vi "VPD Test Panel.vi"() -> ()   [LabVIEW 2020]
uses:
  Desktop/Vision Point LabVIEW/KYFGLib_lv.lvlib
panel:
  out "Intensity Graph":u16[][](graph)
  out "size(s) 0":i32
  in  "Pixel format":enum16{"Mono8", "Mono10", "Mono12"}(ring)
  in  "Adjust width":bool
  in  "Horizontal Pixel slider":cluster{i64, i64}(slide)={9072, 0} scale=0.0..9072.0
  in  "Height":i64=256
  in  "paramValueName":string
  in  "Boolean":bool=TRUE
  out "paramValue our [Float]":dbl
  out "frame index":i32
  out "buffer size":u64
  out "buffHandle":u32
  in  "Start stream":bool
  in  "Float Value (set)":dbl
  in  "Send command":bool
  in  "Integer Value (set)":i64=1
  out "function return":u32
  out "stringValueOut":string
  out "paramValue out [Int]":i64
  in  "Frame Grabber":bool=TRUE
  in  "Camera":bool
  in  "Set Parameter":string
  in  "Get Parameter":string
  out "Frame Grabber handle":u32=65536 caption="FG handle"
  out "Camera handle":u32
  out "Frame Grabbers":string[](array[string])
  in  "Quit":bool
  out "Last Error":errorcluster
  # "Example Commands:\n\nGet info for device\n0in\n\nGet device status\n0gs\n\nGo to home position (position 0)\n0ho0\n\nGo to position 0\n0ma00000000\n\nGo to position 1\n0ma00000020\n\nGo to position 2\n0ma00000040\n\nGo to position 3\n0ma00000060"
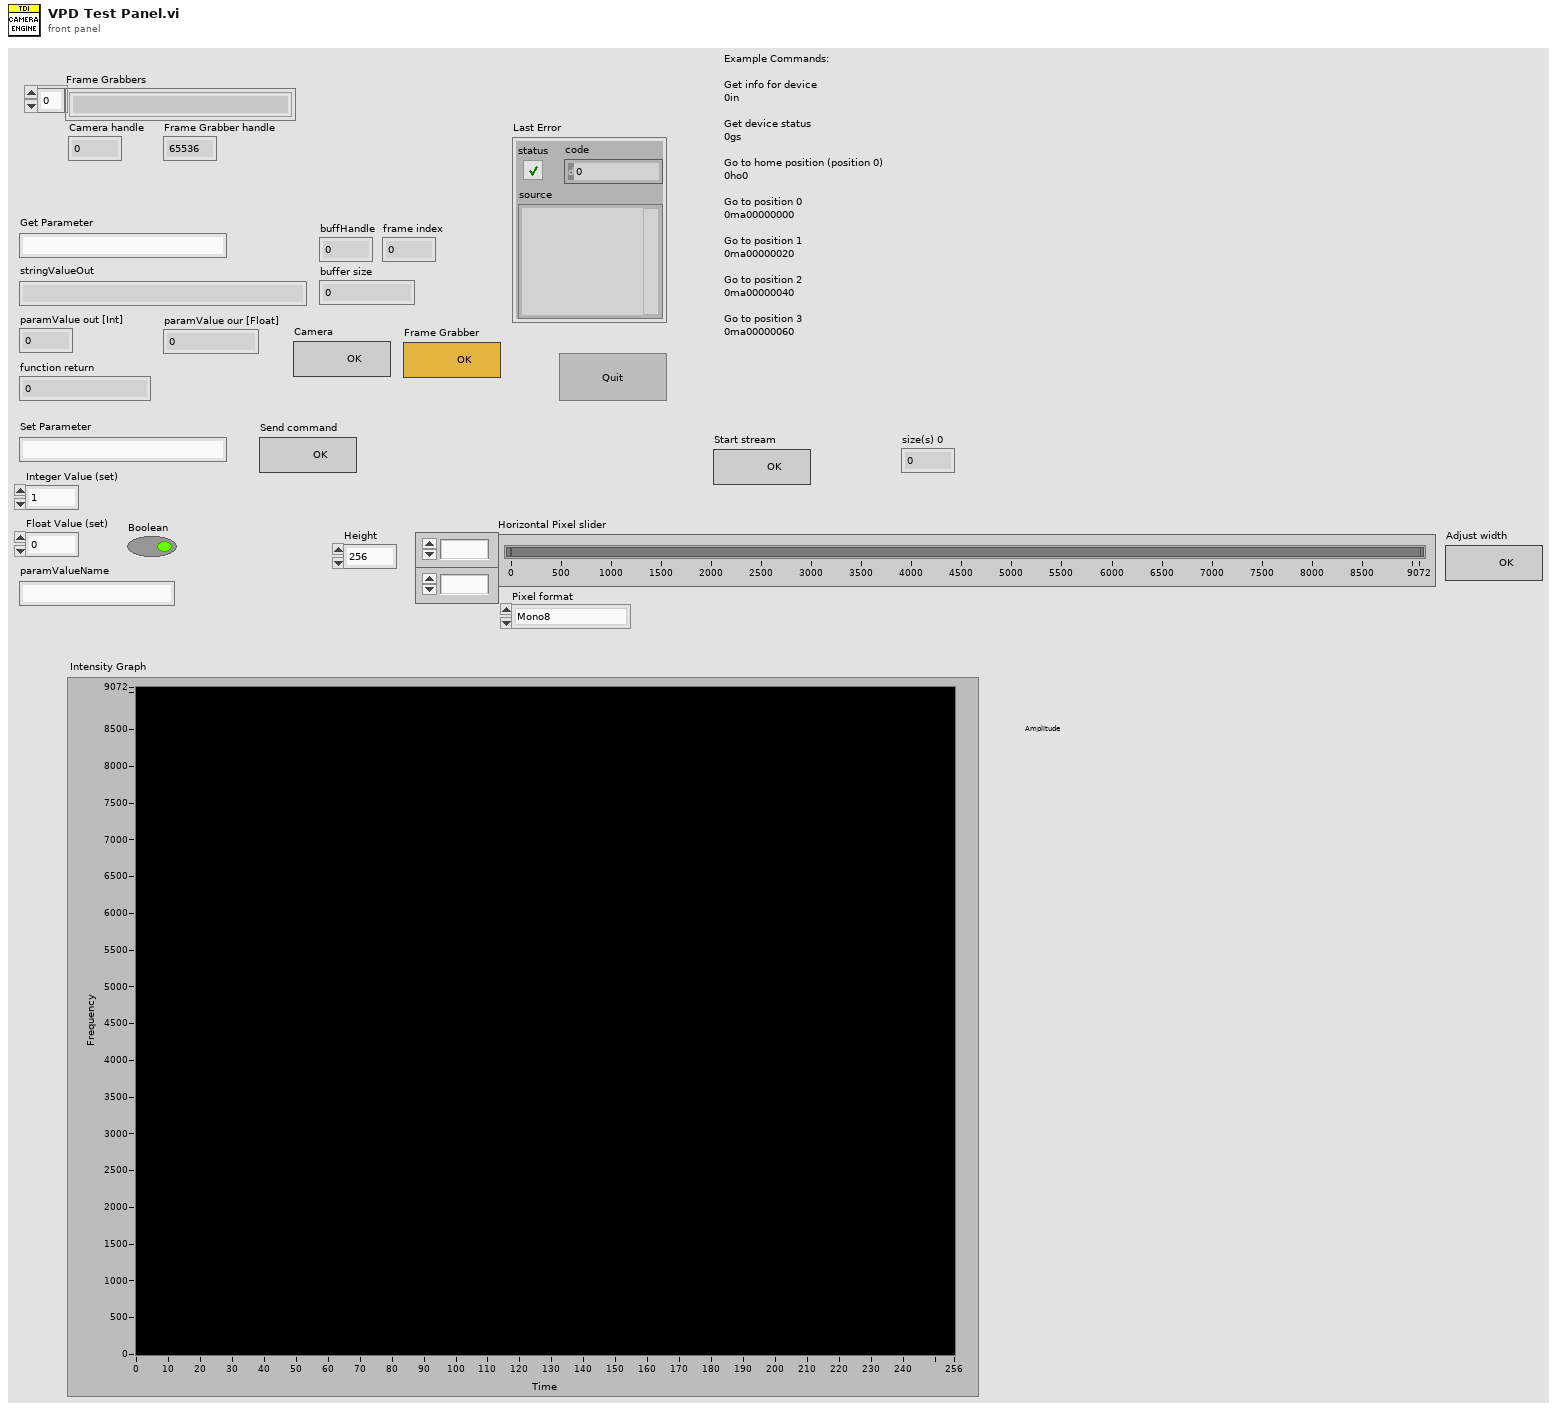
[diagram p1: front panel]
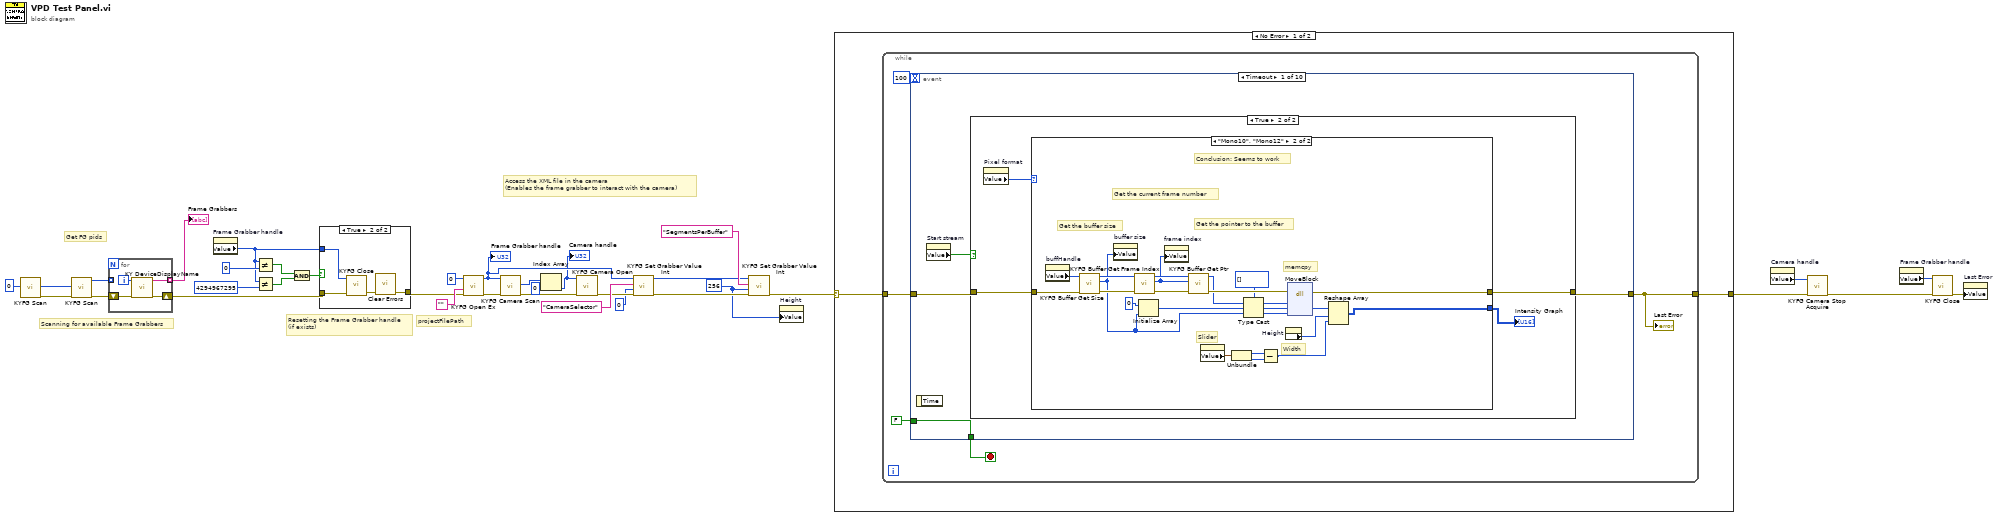
[diagram p0: block diagram]
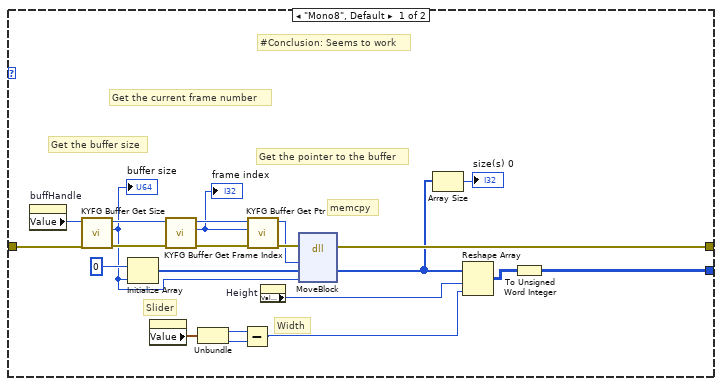
[diagram p3: hidden frame]
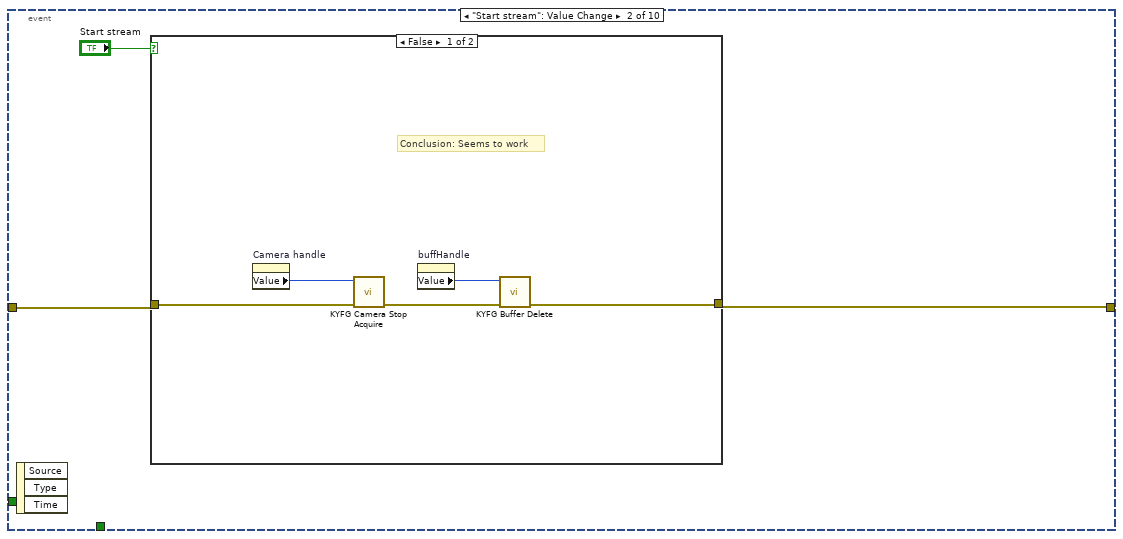
[diagram p4: hidden frame]
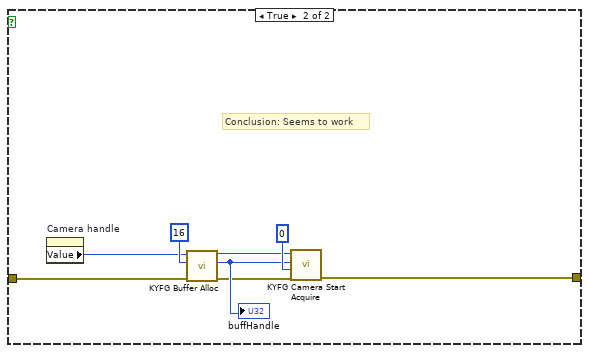
[diagram p5: hidden frame]
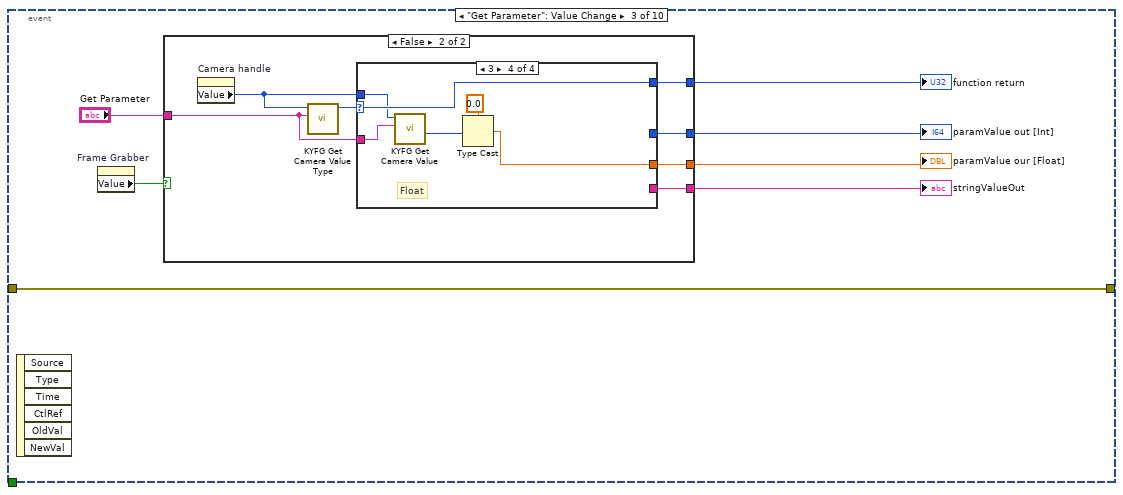
[diagram p6: hidden frame]
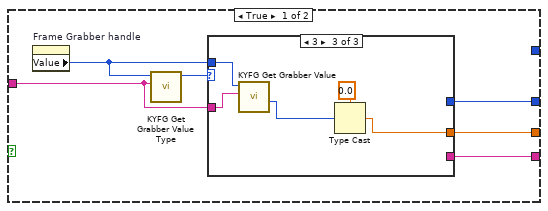
[diagram p7: hidden frame]
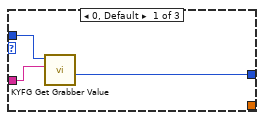
[diagram p8: hidden frame]
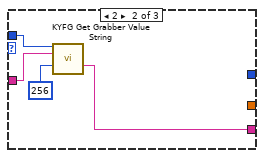
[diagram p9: hidden frame]
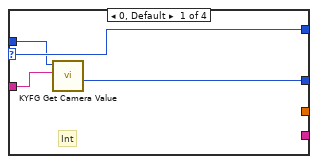
[diagram p10: hidden frame]
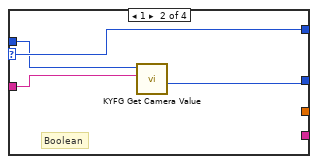
[diagram p11: hidden frame]
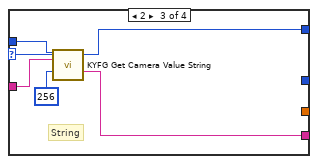
[diagram p12: hidden frame]
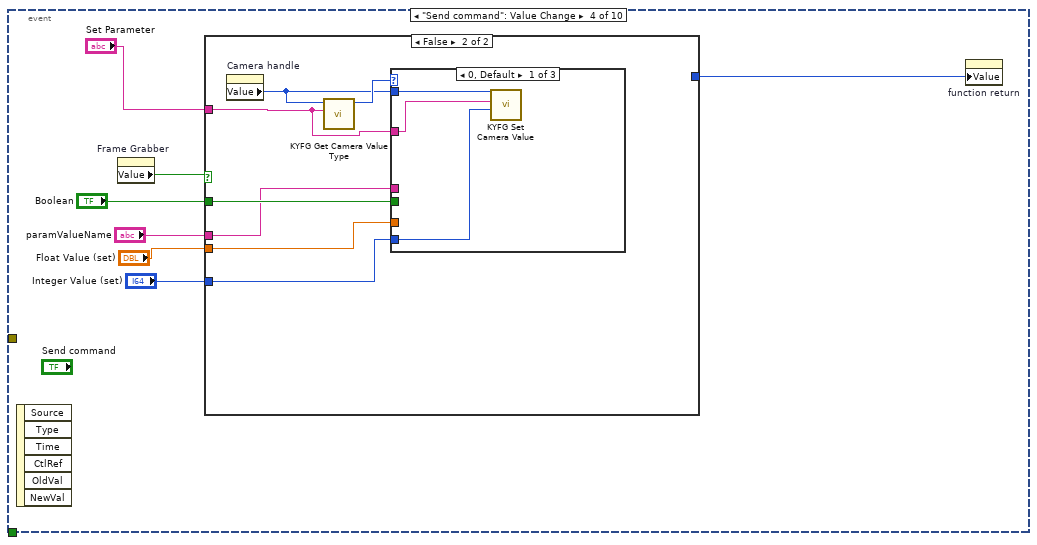
[diagram p13: hidden frame]
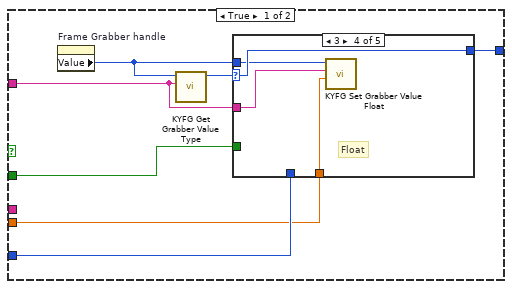
[diagram p14: hidden frame]
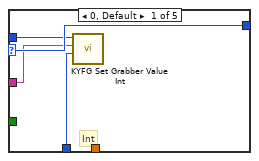
[diagram p15: hidden frame]
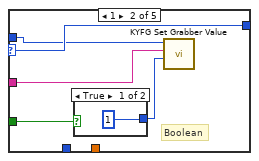
[diagram p16: hidden frame]
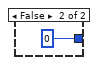
[diagram p17: hidden frame]
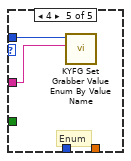
[diagram p19: hidden frame]
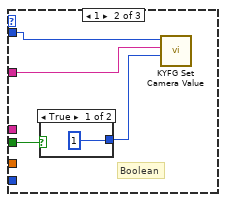
[diagram p20: hidden frame]
diagram:
  w2 = i64 256 ("value")
  # "Access the XML file in the camera\n(Enables the frame grabber to interact with the camera)"
  # "projectFilePath"
  # "Resetting the Frame Grabber handle\n(if exists)"
  # "Scanning for available Frame Grabbers"
  # "Get FG pids"
  n1 = call "KYFG Scan.vi"("count"=0) -> ("error out"=w25:errorcluster, "infosize"=w33:i32)  [unwired: 8 in, 1 out]
  n2 = call "KYFG Scan.vi"("error in (no error)"=w25, "count"=w33) -> ("error out"=w34:errorcluster, "pids_info"=w35:u32[])  [unwired: 7 in, 1 out]
  n3 = for {
    tunnel: w35 -> [_] mode=indexing
    shift-right: [w38] -> w21
    shift-left: w34 -> [w39]
    tunnel: [w36] -> w22 mode=indexing
    i -> [w37]
    n4 = call "KY DeviceDisplayName.vi"("error in (no error)"=w39, "index"=w37) -> ("error out"=w38:errorcluster, "function return"=w36:string)  [unwired: 8 in]
  }
  "Frame Grabbers" <- w22
  n5 = property on="Frame Grabber handle" class="DigNum (strict)"() -> ("Value"=w26:u32)  [unwired: 2 in, 2 out]
  n6 = Not Equal?(x=w26, y=u32 0) -> (x != y?=w32:bool)
  n7 = Not Equal?(x=w26, y=u32 4294967295) -> (x != y?=w31:bool)
  n8 = Compound Arithmetic op=AND(w32, w31) -> (w28:bool)
  n9 = case shown="True" w28 {
    tunnel: [w40 w42] -> w19
    tunnel: w26 -> [_ w44]
    tunnel: w21 -> [w40 w41]
    frame False {
    }
    frame True {
      n10 = call "KYFG Close.vi"("error in (no error)"=w41, "handle"=w44) -> ("error out"=w43:errorcluster)  [unwired: 8 in, 1 out]
      n11 = call <vilib>:"Clear Errors.vi"("error in (no error)"=w43) -> ("error out"=w42:errorcluster)  [unwired: 5 in, 1 out]
    }
  }
  n12 = call "KYFG Open Ex.vi"("error in (no error)"=w19, "projectFile"="", "index"=0) -> ("error out"=w24:errorcluster, "handle"=w8:u32)  [unwired: 7 in]
  "Frame Grabber handle" <- w8
  n13 = call "KYFG Camera Scan.vi"("error in (no error)"=w24, "handle"=w8) -> ("error out"=w10:errorcluster, "camHandleArray"=w18:u32[])  [unwired: 7 in, 1 out]
  n14 = Index Array(array=w18, index=0) -> (element=w4:u32)
  "Camera handle" <- w4
  n15 = call "KYFG Camera Open.vi"("error in (no error)"=w10, "camHandle"=w4) -> ("error out"=w9:errorcluster)  [unwired: 7 in, 2 out]
  n16 = call "KYFG Set Grabber Value Int.vi"("error in (no error)"=w9, "value"=i64 0, "paramName"="CameraSelector", "camHandle"=w8) -> ("error out"=w6:errorcluster, "camHandle out"=w1:u32)  [unwired: 6 in]
  n17 = call "KYFG Set Grabber Value Int.vi"("error in (no error)"=w6, "value"=w2, "paramName"="SegmentsPerBuffer", "camHandle"=w1) -> ("error out"=w5:errorcluster)  [unwired: 6 in, 1 out]
  n18 = property on="Height" class="DigNum (strict)"("Value"=w2) -> ()  [unwired: 2 in, 2 out]
  n19 = case shown="No Error" w5 {
    selector: w5 -> [w46 w320]
    tunnel: [w45 w320] -> w14
    frame No Error {
      n20 = while {
        tunnel: w46 -> [w49]
        tunnel: [w48] -> w45
        stop <- w50 stop-if-true
        n21 = event shown="[0] Timeout" {
          selector: _ -> [_ _ _ _ _ _ _ _ _ _]
          dyn-events: _ -> [_ _ _ _ _ _ _ _ _ _]
          timeout: 100 -> [_ _ _ _ _ _ _ _ _ _]
          tunnel: FALSE -> [w55 _ _ _ _ _ _ _ _ _]
          tunnel: [w55 _ _ _ _ _ _ _ TRUE _] -> w50
          tunnel: w49 -> [w54 w106 w123 _ _ w226 w284 w304 w312 w316]
          tunnel: [w53 w105 w123 _ _ w226 w282 w304 w312 w315] -> w48
          event Timeout {
            n22 = event-data() -> ()  [unwired: 1 in, 1 out]
            n23 = property on="Start stream" class="Bool (strict)"() -> ("Value"=w52:bool)  [unwired: 2 in, 2 out]
            n24 = case shown="True" w52 {
              tunnel: w54 -> [w56 w60]
              tunnel: [w56 w59] -> w53
              frame False {
              }
              frame True {
                n25 = property on="Pixel format" class="Enum (strict)"() -> ("Value"=w58:enum16{"Mono8", "Mono10", "Mono12"})  [unwired: 2 in, 2 out]
                n26 = case shown="\"Mono10\", \"Mono12\"" w58 {
                  tunnel: w60 -> [w82 w104]
                  tunnel: [w70 w95] -> w59
                  tunnel: [w61 w83] -> w57
                  frame "Mono8", Default {
                    # "Width"
                    # "Slider"
                    # "#Conclusion: Seems to work"
                    # "Get the current frame number"
                    # "Get the buffer size"
                    # "Get the pointer to the buffer"
                    # "memcpy"
                    n27 = property on="buffHandle" class="DigNum (strict)"() -> ("Value"=w79:u32)  [unwired: 2 in, 2 out]
                    n28 = call "KYFG Buffer Get Size.vi"("error in (no error)"=w82, "buffHandle"=w79) -> ("error out"=w81:errorcluster, "buffer size"=w71:i32, "buffHandle out"=w78:u32)  [unwired: 7 in]
                    "buffer size" <- w71
                    n29 = Initialize Array(u8 0 ("I32"), w71) -> (w72:u8[])
                    n30 = property on="Horizontal Pixel slider" class="Slide (strict)"() -> ("Value"=w68:cluster{i64, i64})  [unwired: 2 in, 2 out]
                    n31 = call "KYFG Buffer Get Frame Index.vi"("error in (no error)"=w81, "buffHandle"=w78) -> ("error out"=w80:errorcluster, "frame index"=w75:i32, "buffHandle out"=w77:u32)  [unwired: 7 in]
                    "frame index" <- w75
                    n32 = Unbundle(w68) -> (w67:i64, w66:i64)
                    n33 = Subtract(x=w67, y=w66) -> (x-y=w65:i64)
                    n34 = call "KYFG Buffer Get Ptr.vi"("error in (no error)"=w80, "frame"=w75, "buffHandle"=w77) -> ("error out"=w74:errorcluster, "buffer data"=w73:u64)  [unwired: 7 in]
                    n35 = property on="Height" class="DigNum (strict)"() -> ("Value"=w69:i64)  [unwired: 2 in, 2 out]
                    n36 = dll-call lib="LabVIEW" fn="MoveBlock"(error in=w74, "src"=w73, "dst"=w72, "size"=w71) -> (error out=w70:errorcluster, "dst"=w64:u8[])  [unwired: 5 in, 1 out]
                    n37 = Array Size(array=w64) -> (size(s)=→"size(s) 0":i32)
                    n38 = Reshape Array(w64, w69, w65) -> (w62:u8[][])
                    n39 = To Unsigned Word Integer(number=w62) -> (unsigned 16bit integer=w61:u16[][])
                  }
                  frame "Mono10", "Mono12" {
                    # "Width"
                    # "Slider"
                    # "Conclusion: Seems to work"
                    # "Get the current frame number"
                    # "Get the buffer size"
                    # "Get the pointer to the buffer"
                    # "memcpy"
                    n40 = property on="buffHandle" class="DigNum (strict)"() -> ("Value"=w101:u32)  [unwired: 2 in, 2 out]
                    n41 = call "KYFG Buffer Get Size.vi"("error in (no error)"=w104, "buffHandle"=w101) -> ("error out"=w103:errorcluster, "buffer size"=w88:i32, "buffHandle out"=w100:u32)  [unwired: 7 in]
                    n42 = property on="buffer size" class="DigNum (strict)"("Value"=w88) -> ()  [unwired: 2 in, 2 out]
                    n43 = call "KYFG Buffer Get Frame Index.vi"("error in (no error)"=w103, "buffHandle"=w100) -> ("error out"=w102:errorcluster, "frame index"=w89:i32, "buffHandle out"=w99:u32)  [unwired: 7 in]
                    n44 = Initialize Array(u8 0 ("I32"), w88) -> (w86:u8[])
                    n45 = property on="frame index" class="DigNum (strict)"("Value"=w89) -> ()  [unwired: 2 in, 2 out]
                    n46 = call "KYFG Buffer Get Ptr.vi"("error in (no error)"=w102, "frame"=w89, "buffHandle"=w99) -> ("error out"=w97:errorcluster, "buffer data"=w96:u64)  [unwired: 7 in]
                    n47 = property on="Horizontal Pixel slider" class="Slide (strict)"() -> ("Value"=w93:cluster{i64, i64})  [unwired: 2 in, 2 out]
                    n48 = Unbundle(w93) -> (w92:i64, w91:i64)
                    n49 = Type Cast(type=u16[] [] ("initialized array"), x=w86) -> (*(type *) &x=w85:u16[])
                    n50 = Subtract(x=w92, y=w91) -> (x-y=w90:i64)
                    n51 = property on="Height" class="DigNum (strict)"() -> ("Value"=w94:i64)  [unwired: 2 in, 2 out]
                    n52 = dll-call lib="LabVIEW" fn="MoveBlock"(error in=w97, "src"=w96, "dst"=w85, "size"=w88) -> (error out=w95:errorcluster, "dst"=w87:u16[])  [unwired: 5 in, 1 out]
                    n53 = Reshape Array(w87, w94, w90) -> (w83:u16[][])
                  }
                }
                "Intensity Graph" <- w57
              }
            }
          }
          event "Start stream": Value Change {
            n54 = event-data() -> ()  [unwired: 1 in, 3 out]
            n55 = case shown="False" "Start stream" {
              tunnel: w106 -> [w112 w114]
              tunnel: [w110 w113] -> w105
              frame False {
                # "Conclusion: Seems to work"
                n56 = property on="Camera handle" class="DigNum (strict)"() -> ("Value"=w109:u32)  [unwired: 2 in, 2 out]
                n57 = call "KYFG Camera Stop Acquire.vi"("error in (no error)"=w112, "camHandle"=w109) -> ("error out"=w111:errorcluster)  [unwired: 8 in, 1 out]
                n58 = property on="buffHandle" class="DigNum (strict)"() -> ("Value"=w108:u32)  [unwired: 2 in, 2 out]
                n59 = call "KYFG Buffer Delete.vi"("error in (no error)"=w111, "streamHandle"=w108) -> ("error out"=w110:errorcluster)  [unwired: 9 in]
              }
              frame True {
                # "Conclusion: Seems to work"
                n60 = property on="Camera handle" class="DigNum (strict)"() -> ("Value"=w115:u32)  [unwired: 2 in, 2 out]
                n61 = call "KYFG Buffer Alloc.vi"("error in (no error)"=w114, "frames"=u32 16, "camHandle"=w115) -> ("error out"=w116:errorcluster, "buffHandle"=w117:u32, "camHandle out"=w118:u32)  [unwired: 6 in]
                "buffHandle" <- w117
                n62 = call "KYFG Camera Start Acquire.vi"("error in (no error)"=w116, "frames"=u32 0, "buffHandle"=w117, "camHandle"=w118) -> ("error out"=w113:errorcluster)  [unwired: 5 in, 2 out]
              }
            }
          }
          event "Get Parameter": Value Change {
            n63 = event-data() -> ()  [unwired: 1 in, 6 out]
            n64 = property on="Frame Grabber" class="Bool (strict)"() -> ("Value"=w127:bool)  [unwired: 2 in, 2 out]
            n65 = case shown="False" w127 {
              tunnel: "Get Parameter" -> [w131 w147]
              tunnel: [w130 w152] -> w121
              tunnel: [w129 w151] -> w125
              tunnel: [_ w150] -> w124
              tunnel: [w128 w146] -> w122
              frame True {
                n66 = property on="Frame Grabber handle" class="DigNum (strict)"() -> ("Value"=w132:u32)  [unwired: 2 in, 2 out]
                n67 = call "KYFG Get Grabber Value Type.vi"("paramName"=w131, "handle"=w132) -> ("function return"=w133:u32)  [unwired: 8 in, 1 out]
                n68 = case shown="3" w133 {
                  tunnel: w132 -> [w136 w139 w145]
                  tunnel: w131 -> [w135 w138 w144]
                  tunnel: [w134 _ _] -> w130
                  tunnel: [_ w137 _] -> w129
                  tunnel: [_ _ w141] -> w128
                  frame 0, Default {
                    n69 = call "KYFG Get Grabber Value.vi"("paramName"=w135, "handle"=w136) -> ("paramValue out"=w134:i64)  [unwired: 7 in, 2 out]
                  }
                  frame 2 {
                    n70 = call "KYFG Get Grabber Value String.vi"("handle"=w139, "paramName"=w138, "stringSize"=u32 256) -> ("stringValueOut"=w137:string)  [unwired: 10 in, 2 out]
                  }
                  frame 3 {
                    n71 = call "KYFG Get Grabber Value.vi"("paramName"=w144, "handle"=w145) -> ("paramValue out"=w142:i64)  [unwired: 7 in, 2 out]
                    n72 = Type Cast(type=0.0, x=w142) -> (*(type *) &x=w141:dbl)
                  }
                }
              }
              frame False {
                n73 = property on="Camera handle" class="DigNum (strict)"() -> ("Value"=w148:u32)  [unwired: 2 in, 2 out]
                n74 = call "KYFG Get Camera Value Type.vi"("paramName"=w147, "camHandle"=w148) -> ("function return"=w149:u32)  [unwired: 8 in, 1 out]
                n75 = case shown="3" w149 {
                  selector: w149 -> [w156 w160 w165 w171]
                  tunnel: w148 -> [w153 w158 w162 w169]
                  tunnel: w147 -> [w154 w159 w163 w170]
                  tunnel: [w155 w157 _ _] -> w152
                  tunnel: [_ _ w164 _] -> w151
                  tunnel: [w156 w160 w165 w171] -> w150
                  tunnel: [_ _ _ w166] -> w146
                  frame 0, Default {
                    # "Int"
                    n76 = call "KYFG Get Camera Value.vi"("paramName"=w154, "camHandle"=w153) -> ("paramValue"=w155:i64)  [unwired: 7 in, 2 out]
                  }
                  frame 1 {
                    # "Boolean"
                    n77 = call "KYFG Get Camera Value.vi"("paramName"=w159, "camHandle"=w158) -> ("paramValue"=w157:i64)  [unwired: 7 in, 2 out]
                  }
                  frame 2 {
                    # "String"
                    n78 = call "KYFG Get Camera Value String.vi"("camHandle"=w162, "paramName"=w163, "stringSize"=u32 256) -> ("stringValueOut"=w164:string)  [unwired: 10 in, 2 out]
                  }
                  frame 3 {
                    # "Float"
                    n79 = call "KYFG Get Camera Value.vi"("paramName"=w170, "camHandle"=w169) -> ("paramValue"=w168:i64)  [unwired: 7 in, 2 out]
                    n80 = Type Cast(type=0.0, x=w168) -> (*(type *) &x=w166:dbl)
                  }
                }
              }
            }
            "stringValueOut" <- w125
            "function return" <- w124
            "paramValue our [Float]" <- w122
            "paramValue out [Int]" <- w121
          }
          event "Send command": Value Change {
            n81 = event-data() -> ()  [unwired: 1 in, 6 out]
            n82 = property on="Frame Grabber" class="Bool (strict)"() -> ("Value"=w177:bool)  [unwired: 2 in, 2 out]
            n83 = case shown="False" w177 {
              tunnel: "Set Parameter" -> [w183 w208]
              tunnel: [w182 _] -> w176
              tunnel: "Integer Value (set)" -> [w181 w207]
              tunnel: "Boolean" -> [w180 w205]
              tunnel: "Float Value (set)" -> [w179 w206]
              tunnel: "paramValueName" -> [_ w204]
              frame True {
                n84 = property on="Frame Grabber handle" class="DigNum (strict)"() -> ("Value"=w184:u32)  [unwired: 2 in, 2 out]
                n85 = call "KYFG Get Grabber Value Type.vi"("paramName"=w183, "handle"=w184) -> ("function return"=w185:u32)  [unwired: 8 in, 1 out]
                n86 = case shown="3" w185 {
                  selector: w185 -> [w189 w194 w197 w201 _]
                  tunnel: w184 -> [w188 w190 _ w200 w203]
                  tunnel: w183 -> [w187 w191 _ w199 w202]
                  tunnel: [w189 w194 w197 w201 _] -> w182
                  tunnel: w181 -> [w186 _ _ _ _]
                  tunnel: w180 -> [_ w193 _ _ _]
                  tunnel: w179 -> [_ _ _ w198 _]
                  frame 0, Default {
                    # "Int"
                    n87 = call "KYFG Set Grabber Value Int.vi"("value"=w186, "paramName"=w187, "camHandle"=w188) -> ()  [unwired: 7 in, 2 out]
                  }
                  frame 1 {
                    # "Boolean"
                    n88 = case shown="True" w193 {
                      tunnel: [i64 1 0] -> w192
                      frame True {
                      }
                      frame False {
                      }
                    }
                    n89 = call "KYFG Set Grabber Value.vi"("paramValue"=w192, "paramName"=w191, "handle"=w190) -> ()  [unwired: 6 in, 3 out]
                  }
                  frame 2 {
                    # "String"
                  }
                  frame 3 {
                    # "Float"
                    n90 = call "KYFG Set Grabber Value Float.vi"("value"=w198, "paramName"=w199, "handle"=w200) -> ()  [unwired: 7 in, 2 out]
                  }
                  frame 4 {
                    # "Enum"
                    n91 = call "KYFG Set Grabber Value Enum By Value Name.vi"("paramName"=w202, "handle"=w203) -> ()  [unwired: 8 in, 2 out]
                  }
                }
              }
              frame False {
                n92 = property on="Camera handle" class="DigNum (strict)"() -> ("Value"=w209:u32)  [unwired: 2 in, 2 out]
                n93 = call "KYFG Get Camera Value Type.vi"("paramName"=w208, "camHandle"=w209) -> ("function return"=w210:u32)  [unwired: 8 in, 1 out]
                n94 = case shown="0, Default" w210 {
                  tunnel: w209 -> [w213 w216 w222]
                  tunnel: w208 -> [w212 w215 w221]
                  tunnel: w207 -> [w211 _ _]
                  tunnel: w206 -> [_ _ w220]
                  tunnel: w205 -> [_ w217 _]
                  tunnel: w204 -> [_ _ _]
                  frame 0, Default {
                    n95 = call "KYFG Set Camera Value.vi"("paramValue"=w211, "paramName"=w212, "camHandle"=w213) -> ()  [unwired: 7 in, 2 out]
                  }
                  frame 1 {
                    # "Boolean"
                    n96 = case shown="True" w217 {
                      tunnel: [i64 1 0] -> w214
                      frame True {
                      }
                      frame False {
                      }
                    }
                    n97 = call "KYFG Set Camera Value.vi"("paramValue"=w214, "paramName"=w215, "camHandle"=w216) -> ()  [unwired: 7 in, 2 out]
                  }
                  frame 3 {
                    n98 = call "KYFG Set Camera Value Float.vi"("value"=w220, "paramName"=w221, "camHandle"=w222) -> ()  [unwired: 7 in, 2 out]
                  }
                }
              }
            }
            n99 = property on="function return" class="DigNum (strict)"("Value"=w176) -> ()  [unwired: 2 in, 2 out]
          }
          event "Height": Value Change {
            n100 = event-data() -> ()  [unwired: 1 in, 6 out]
            n101 = property on="Frame Grabber handle" class="DigNum (strict)"() -> ("Value"=w224:u32)  [unwired: 2 in, 2 out]
            n102 = call "KYFG Set Grabber Value Int.vi"("value"="Height", "paramName"="SegmentsPerBuffer", "camHandle"=w224) -> ()  [unwired: 7 in, 2 out]
          }
          event "Horizontal Pixel slider": Value Change {
            n103 = event-data() -> ()  [unwired: 1 in, 6 out]
            n104 = for {
              N: 3 -> [_]
              shift-right: [w231] -> w228
              shift-left: "Horizontal Pixel slider" -> [w232]
              i -> [w230]
              n105 = case shown="0, Default" w230 {
                tunnel: w232 -> [w236 w249 w279]
                tunnel: [w233 w248 w272] -> w231
                frame 0, Default {
                  # "First, check if upper boundary is greater than lower boundary"
                  # "lower"
                  # "upper"
                  n106 = Unbundle(w236) -> (w235:i64, w234:i64)
                  n107 = Greater?(x=w235, y=w234) -> (0:w237:bool)
                  n108 = case shown="False" w237 {
                    tunnel: w236 -> [w241 w242]
                    tunnel: w235 -> [w238 _]
                    tunnel: w234 -> [w240 _]
                    tunnel: [w239 w242] -> w233
                    frame False {
                      n109 = Bundle(cluster=w241, w240, w238) -> (w239:cluster{i64, i64})
                    }
                    frame True {
                    }
                  }
                }
                frame 1 {
                  w244 = i64 0 ("lower limit")
                  # "Check that the width and offset\nis within the accepted range.\nWidth range: 256-9072\nOffset range: 0 or integer multiple of 16"
                  # "upper"
                  # "lower"
                  n110 = Unbundle(w249) -> (w254:i64, w247:i64)
                  n111 = Quotient & Remainder(x=w247, y=i64 16) -> (x-y*floor(x/y)=w245:i64)  [unwired: 1 out]
                  n112 = In Range and Coerce(upper limit=i64 256, x=w254, lower limit=w244) -> (In Range?=w252:bool)  [unwired: 1 out]
                  n113 = Equal?(x=w244, y=w245) -> (x = y?=w243:bool)
                  n114 = Build Array(w252, w243) -> (w251:bool[])
                  n115 = Boolean Array To Number(Boolean array=w251) -> (number=w250:u8)
                  n116 = case shown="2" w250 {
                    tunnel: w249 -> [w255 w268 _]
                    tunnel: [w255 w258 cluster{i64, i64} {256, 0} ("Horizontal Pixel slider")] -> w248
                    frame 0, Default {
                    }
                    frame 2 {
                      w263 = i64 256 ("y")
                      n117 = Unbundle(w268) -> (w260:i64, w267:i64)
                      n118 = Divide(x=w267, y=w263) -> (x/y=w266:dbl)
                      n119 = Round To Nearest(number=w266) -> (nearest integer value=w265:dbl)
                      n120 = To Quad Integer(1:w265) -> (0:w264:i64)
                      n121 = Multiply(x=w264, y=w263) -> (x*y=w257:i64)
                      n122 = Add(x=i64 16, y=w260) -> (x+y=w261:i64)
                      n123 = Less Or Equal?(x=w260, y=w257) -> (x <= y?=w262:bool)
                      n124 = Select(t=w261, s=w262, f=w260) -> (s? t:f=w256:i64)
                      n125 = Bundle(w256, w257) -> (w258:cluster{i64, i64})  [unwired: 1 in]
                    }
                    frame 3 {
                    }
                  }
                }
                frame 2 {
                  n126 = Unbundle(w279) -> (w273:i64, w276:i64)
                  n127 = In Range and Coerce(upper limit=i64 9072, x=w276, lower limit=i64 0) -> (coerced(x)=w270:i64)  [unwired: 1 out]
                  n128 = In Range and Coerce(upper limit=i64 9072, x=w273, lower limit=i64 0) -> (coerced(x)=w271:i64)  [unwired: 1 out]
                  n129 = Bundle("upper limit"=w271, "upper limit"=w270) -> (w272:cluster{"upper limit":i64, "upper limit":i64})  [unwired: 1 in]
                }
              }
            }
            n130 = property on="Horizontal Pixel slider" class="Slide (strict)"("Value"=w228) -> ()  [unwired: 2 in, 2 out]
          }
          event "Adjust width": Value Change {
            n131 = event-data() -> ()  [unwired: 1 in, 6 out]
            n132 = property on="Start stream" class="Bool (strict)"() -> ("Value"=w286:bool)  [unwired: 2 in, 2 out]
            n133 = case shown="False" w286 {
              tunnel: "Adjust width" -> [w291 _]
              tunnel: w284 -> [w290 w303]
              tunnel: [w289 w303] -> w281
              frame False {
                n134 = case shown="True" w291 {
                  tunnel: w290 -> [w292 w298]
                  tunnel: [w292 w293] -> w289
                  frame False {
                  }
                  frame True {
                    n135 = property on="Horizontal Pixel slider" class="Slide (strict)"() -> ("Value"=w302:cluster{i64, i64})  [unwired: 2 in, 2 out]
                    n136 = property on="Camera handle" class="DigNum (strict)"() -> ("Value"=w301:u32)  [unwired: 2 in, 2 out]
                    n137 = Unbundle(w302) -> (w294:i64, w299:i64)
                    n138 = call "KYFG Set Camera Value.vi"("error in (no error)"=w298, "paramValue"=w299, "paramName"="OffsetX", "camHandle"=w301) -> ("error out"=w297:errorcluster, "camHandle out"=w296:u32)  [unwired: 6 in]
                    n139 = call "KYFG Set Camera Value.vi"("error in (no error)"=w297, "paramValue"=w294, "paramName"="Width", "camHandle"=w296) -> ("error out"=w293:errorcluster)  [unwired: 6 in, 1 out]
                  }
                }
              }
              frame True {
              }
            }
            n140 = flat-sequence {
              tunnel: w281 -> [w288]
              tunnel: [w288] -> w280
              frame #0 {
                n141 = Wait (ms)(milliseconds to wait=u32 250) -> ()  [unwired: 1 out]
              }
            }
            n142 = property on="Adjust width" class="Bool (strict)"(error in=w280, "Value"=FALSE ("Adjust width")) -> (error out=w282:errorcluster)  [unwired: 1 in, 1 out]
          }
          event "Camera", "Frame Grabber": Value Change {
            n143 = event-data() -> ("CtlRef"=w306:refnum<vi>)  [unwired: 1 in]
            n144 = property class="Bool (strict)"(reference=w306) -> ("Label.Text"=w305:string)  [unwired: 1 in, 2 out]
            n145 = case shown="\"Camera\"" w305 {
              frame "0", Default {
              }
              frame "Camera" {
                n146 = Not(x="Camera") -> (.not. x?=w307:bool)
                n147 = property on="Frame Grabber" class="Bool (strict)"("Value"=w307) -> ()  [unwired: 2 in, 2 out]
              }
              frame "Frame Grabber" {
                n148 = Not(x="Frame Grabber") -> (.not. x?=w309:bool)
                n149 = property on="Camera" class="Bool (strict)"("Value"=w309) -> ()  [unwired: 2 in, 2 out]
              }
            }
          }
          event "Quit": Value Change {
            n150 = event-data() -> ()  [unwired: 1 in, 1 out]
          }
          event "Pixel format": Value Change {
            n151 = event-data() -> ()  [unwired: 1 in, 6 out]
            n152 = property on="Camera handle" class="DigNum (strict)"() -> ("Value"=w317:u32)  [unwired: 2 in, 2 out]
            n153 = Format Into String(format string="%s", "Pixel format") -> (resulting string=w314:string)  [unwired: 2 in, 1 out]
            n154 = call "KYFG Set Camera Value Enum By Value Name.vi"("error in (no error)"=w316, "paramValueName"=w314, "paramName"="PixelFormat", "camHandle"=w317) -> ("error out"=w315:errorcluster)  [unwired: 6 in, 1 out]
          }
        }
        "Last Error" <- w48
      }
    }
    frame Error {
    }
  }
  n155 = property on="Camera handle" class="DigNum (strict)"() -> ("Value"=w12:u32)  [unwired: 2 in, 2 out]
  n156 = call "KYFG Camera Stop Acquire.vi"("error in (no error)"=w14, "camHandle"=w12) -> ("error out"=w13:errorcluster)  [unwired: 8 in, 1 out]
  n157 = property on="Frame Grabber handle" class="DigNum (strict)"() -> ("Value"=w16:u32)  [unwired: 2 in, 2 out]
  n158 = call "KYFG Close.vi"("error in (no error)"=w13, "handle"=w16) -> ("error out"=w15:errorcluster)  [unwired: 8 in, 1 out]
  n159 = property on="Last Error" class="Clust (strict)"("Value"=w15) -> ()  [unwired: 2 in, 2 out]
